vi "Recipes Dequeue.vi"(8 "error in (no error)":errorcluster, 11 "Queue in":refnum<queue>) -> (0 "error out":errorcluster, 1 "Data":variant, 2 "State":T1, 3 "Queue out":refnum<queue>)   [LabVIEW 2017, in "Recipes.lvclass"]
uses:
  Recipes.lvclass
  Type Defs/Recipes State.ctl
  Recipes.lvclass/Recipes.ctl
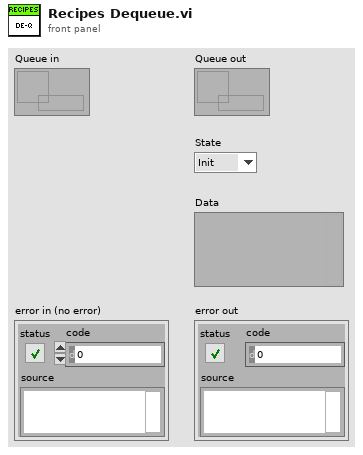
[diagram p1: front panel]
types:
  T1 = typedef "Recipes.lvclass/Recipes State.ctl" = enum16{"Init", "Update List", "Create", "Send", "Load", "Save", "Idle", "Error", "Shutdown"}
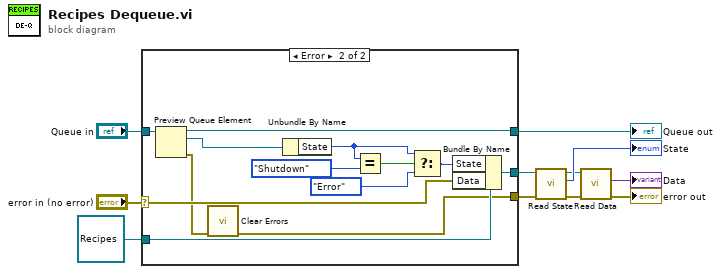
[diagram p0: block diagram]
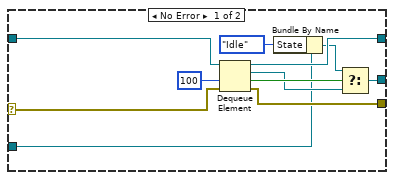
[diagram p2: hidden frame]
diagram:
  n1 = case shown="Error" "error in (no error)" {
    selector: "error in (no error)" -> [w21 w34]
    tunnel: "Queue in" -> [w22 w26]
    tunnel: [w15 w35] -> w3
    tunnel: [w20 w27] -> w1
    tunnel: [w19 w28] -> w2
    tunnel: refnum<class "Recipes.lvclass"> refnum ("Expansion.lvclass") -> [w12 w33]
    frame No Error {
      n2 = Dequeue Element(queue=w22, timeout in ms (-1)=100, error in (no error)=w21) -> (queue out=w20:refnum<queue>, element=w16:refnum<class "Recipes.lvclass">, timed out?=w17:bool, error out=w19:errorcluster)
      n3 = Bundle By Name(cluster=w12, "State"=Recipes_State."Idle") -> (w14:refnum<class "Recipes.lvclass">)
      n4 = Select(t=w14, s=w17, f=w16) -> (s? t:f=w15:refnum<class "Recipes.lvclass">)
    }
    frame Error {
      n5 = Preview Queue Element(queue=w26) -> (queue out=w27:refnum<queue>, element=w32:refnum<class "Recipes.lvclass">, error out=w31:errorcluster)  [unwired: 2 in, 1 out]
      n6 = call <vilib>:"Clear Errors.vi"("error in (no error)"=w31) -> ("error out"=w28:errorcluster)  [unwired: 5 in, 1 out]
      n7 = Unbundle By Name(w32) -> ("State"=w29:T1)
      n8 = Equal?(x=w29, y=Recipes_State."Shutdown") -> (x = y?=w30:bool)
      n9 = Select(t=w29, s=w30, f=Recipes_State."Error" ("State")) -> (s? t:f=w23:T1)
      n10 = Bundle By Name(cluster=w33, "State"=w23, "Data"=w34) -> (w35:refnum<class "Recipes.lvclass">)
    }
  }
  "Queue out" <- w1
  n11 = call "Read State.vi"("error in (no error)"=w2, "Expansion in"=w3) -> ("error out"=w8:errorcluster, "State"=→"State":T1, "Expansion out"=w10:refnum<class "Recipes.lvclass">)  [unwired: 7 in]
  n12 = call "Read Data.vi"("error in (no error)"=w8, "Expansion in"=w10) -> ("error out"=→"error out":errorcluster, "Data"=→"Data":variant)  [unwired: 7 in, 1 out]
